vi "SavePanel.vi"(8 "error in":errorcluster) -> (0 "error out":errorcluster, 3 "Chaîne":string)   [LabVIEW 2019, in "PhotoLum.lvclass"]
uses:
  PhotoLum.lvclass
panel:
  in  "OtherMat":string caption="Matériaux (autres)"
  in  "Matériaux":u16(ring) items=["AlGaAs", "AlP", "GaAs", "GaN", "Ge", "InP", "Si", "SiGe", "Autres"]
  in  "unit":u16(ring) caption="Unités\nPre-amp." items=["mA/V", "µA/V", "nA/V", "pA/V"]
  in  "Facteur":u16(ring) caption="Facteur Pre-amp." items=["1", "2", "5", "10", "20", "50", "100", "200", "500"]
  in  "Preamp":u16(ring) caption="Pre-amplificateur" items=["Aucun", "SR570 Current Preamp", "SR560 Voltage Preamp"]
  in  "PLaser":dbl=1000.0 caption="Puissance(mW)" min=0.0 step=0.1 format="%#.1f"
  in  "Temp":dbl=1000.0 caption="Température(°K)" min=0.0 step=0.1 format="%#.1f"
  in  "Annuler":bool
  in  "Save":bool
  in  "Autres":string
  in  "Filtre":u16(ring) caption="Filtre Entrée" items=["Aucun", "Mauve", "Jaune 495nm", "Vert", "Orange", "Rouge 665nm", "Rouge 850nm", "SI"]
  in  "LN Cooled":bool
  in  "Échantillon":string
  in  "Excitation":u16(ring) caption="Source d'excitation" items=["HeCd 325nm", "Diode 532nm", "Diode 683nm", "Diode 786nm", "Diode 840nm", "Diode 905nm", "Diode 980nm"]
  in  "Détecteur":u16(ring) items=["PM Hamamatsu R9268", "Détecteur Ge EG&G", "Détecteur Si EG&G", "Détecteur InAs EG&G", "Détecteur InSb EG&G"]
  in  "Réseaux":u16(ring) items=["250nm", "1µm", "4µm", "8µm"]
  in  "2xInput":bool
  in  "OutputSlit":dbl caption="Largeur de fente de sortie (mm)"
  in  "SlitHeight":u16(ring) caption="Hauteur fente d'entrée" items=["2 cm", "1 cm", "2 mm", "Trou haut", "Trou centré", "Trou bas"]
  in  "InputSlit":dbl caption="Largeur de fente d'entrée (mm)"
  # "Paramètres du balayage"
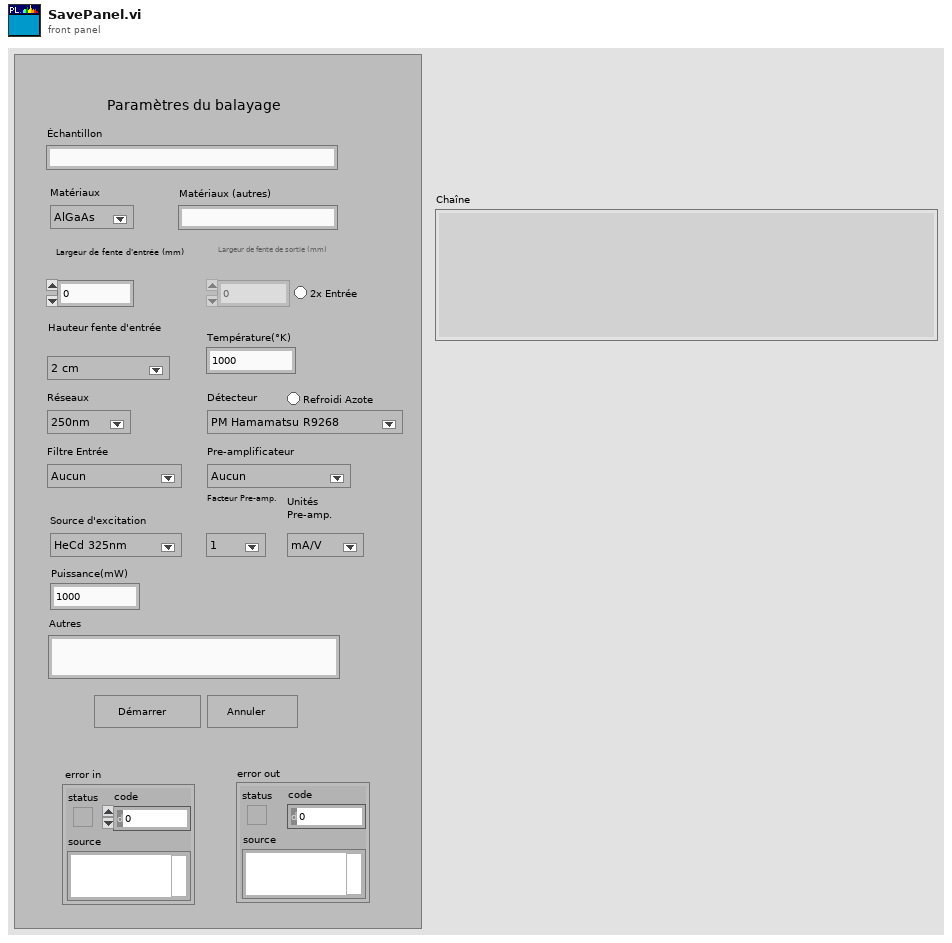
[diagram p1: front panel]
types:
  T1 = enum8{"Enabled", "Disabled", "Disabled and Grayed Out"}
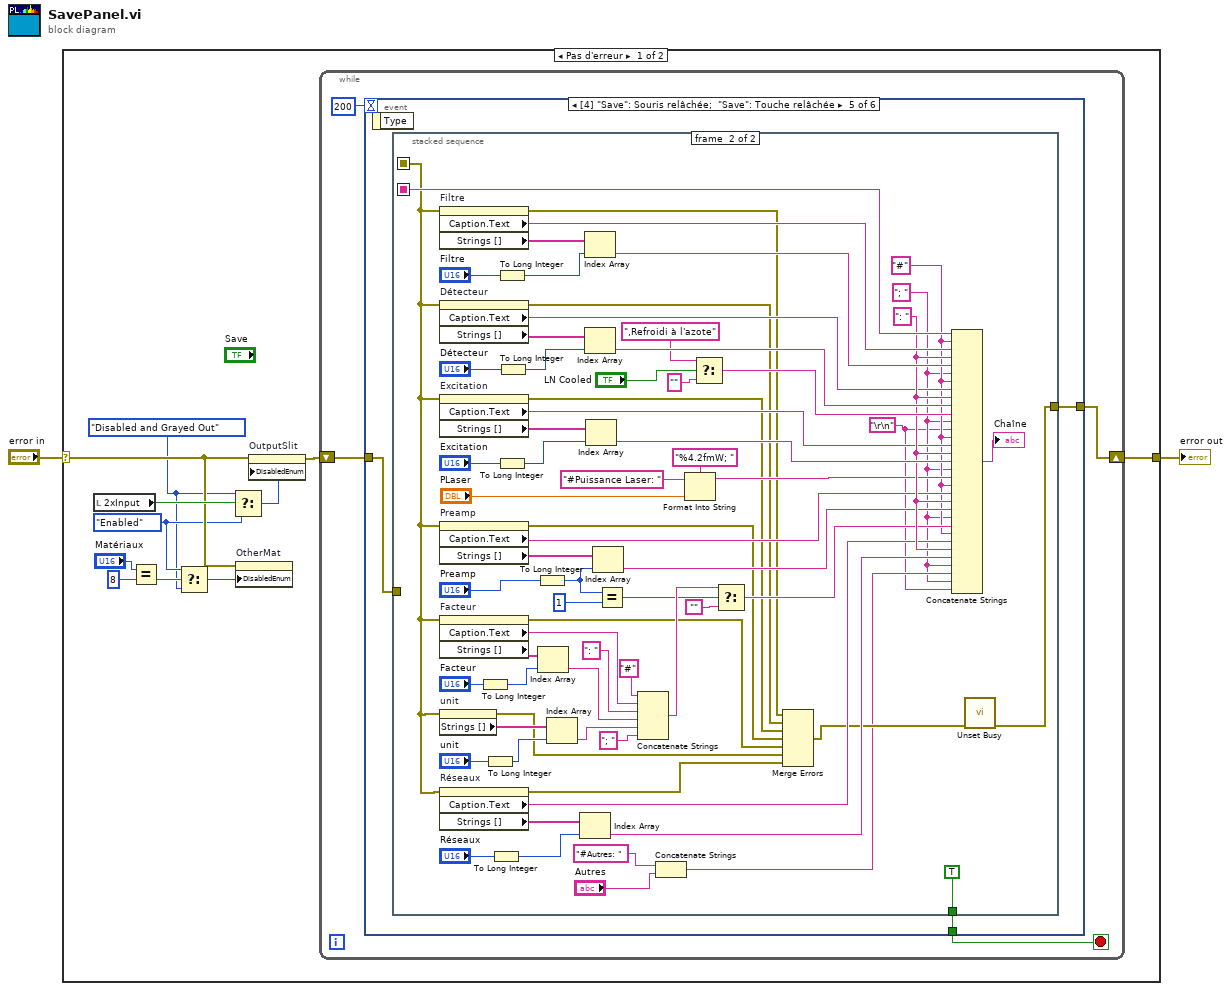
[diagram p0: block diagram]
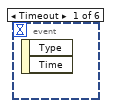
[diagram p2: hidden frame]
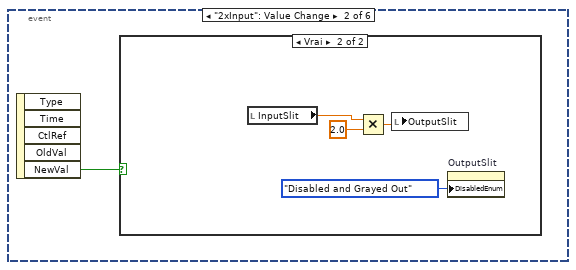
[diagram p3: hidden frame]
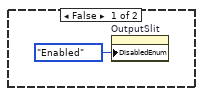
[diagram p4: hidden frame]
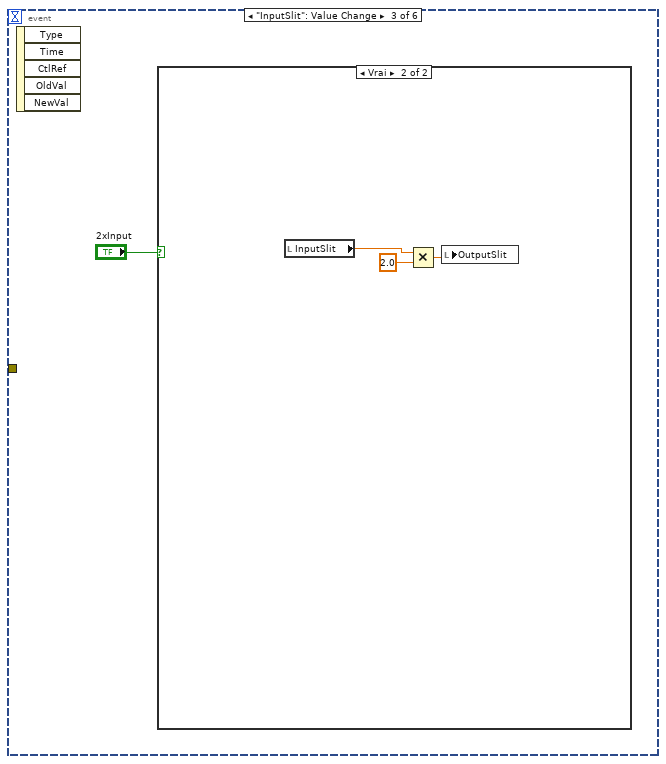
[diagram p5: hidden frame]
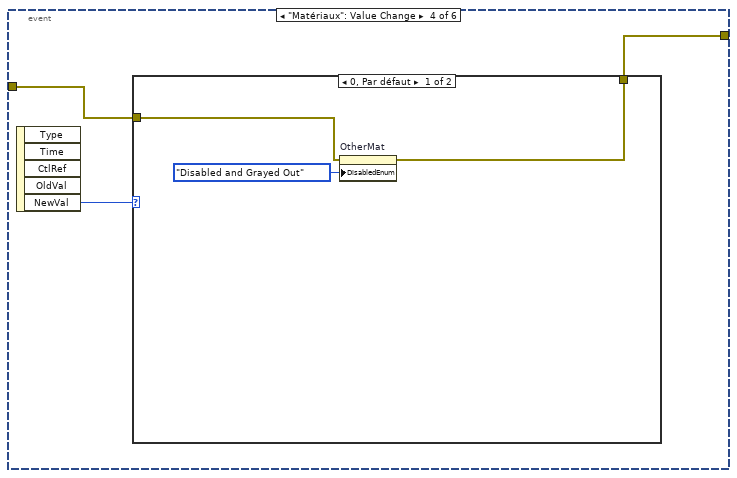
[diagram p7: hidden frame]
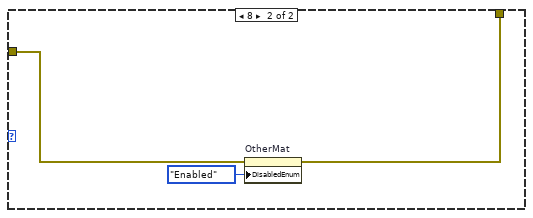
[diagram p8: hidden frame]
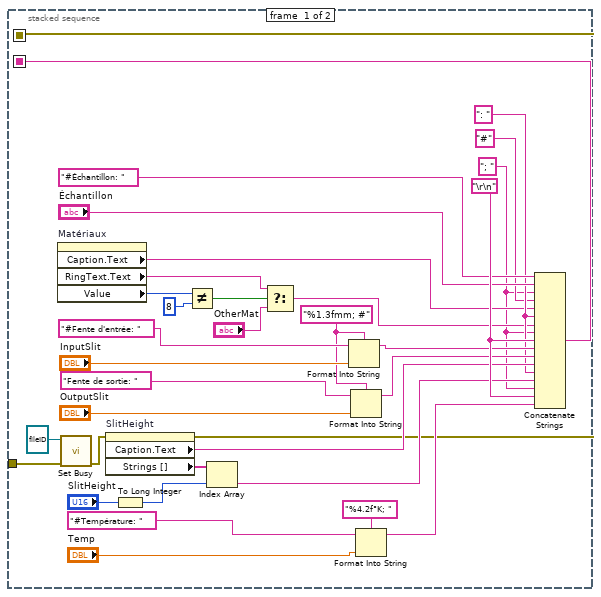
[diagram p9: hidden frame]
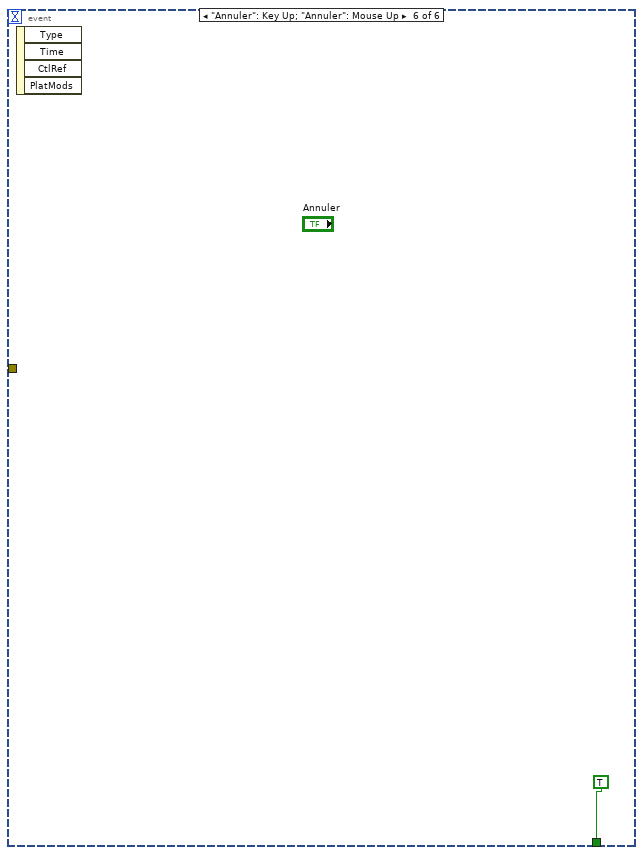
[diagram p10: hidden frame]
diagram:
  n1 = case shown="Pas d'erreur" "error in" {
    selector: "error in" -> [w9 w145]
    tunnel: [w13 w145] -> w2
    frame No Error {
      w4 = T1."Disabled and Grayed Out" ("Désactivé")
      w5 = T1."Enabled" ("Désactivé")
      n2 = local read "2xInput"() -> (w11:bool)
      n3 = Equal?(x="Matériaux", y=u16 8) -> (x = y?=w6:bool)
      n4 = Select(t=w5, s=w6, f=w4) -> (s? t:f=w3:T1)
      n5 = Select(t=w4, s=w11, f=w5) -> (s? t:f=w10:T1)
      n6 = property on="OtherMat" class="Ch"(error in=w9, "DisabledEnum"=w3) -> ()  [unwired: 1 in, 2 out]
      n7 = property on="OutputSlit" class="NumNb (strict)"(error in=w9, "DisabledEnum"=w10) -> (error out=w12:errorcluster)  [unwired: 1 in, 1 out]
      n8 = while {
        shift-right: [w14] -> w13
        shift-left: w12 -> [w15]
        stop <- w16 stop-if-true
        n9 = event shown="[4] \"Save\": Souris relâchée;  \"Save\": Touche relâchée" {
          selector: _ -> [_ _ _ _ _ _]
          dyn-events: _ -> [_ _ _ _ _ _]
          timeout: 200 -> [_ _ _ _ _ _]
          tunnel: [_ _ _ _ w39 TRUE] -> w16
          tunnel: w15 -> [_ _ _ w29 w38 _]
          tunnel: [_ _ _ w28 w37 _] -> w14
          event Timeout {
            n10 = event-data() -> ()  [unwired: 1 in, 2 out]
          }
          event "2xInput": Value Change {
            n11 = event-data() -> ("NewVal"=w18:bool)  [unwired: 1 in, 4 out]
            n12 = case shown="Vrai" w18 {
              frame False {
                n13 = property on="OutputSlit" class="NumNb (strict)"("DisabledEnum"=T1."Enabled" ("Désactivé")) -> ()  [unwired: 2 in, 2 out]
              }
              frame True {
                n14 = local read "InputSlit"() -> (w20:dbl)
                n15 = Multiply(x=w20, y=2.0) -> (x*y=w22:dbl)
                n16 = local write "OutputSlit"(w22) -> ()
                n17 = property on="OutputSlit" class="NumNb (strict)"("DisabledEnum"=T1."Disabled and Grayed Out" ("Désactivé")) -> ()  [unwired: 2 in, 2 out]
              }
            }
          }
          event "InputSlit": Value Change {
            n18 = event-data() -> ()  [unwired: 1 in, 5 out]
            n19 = case shown="Vrai" "2xInput" {
              frame False {
              }
              frame True {
                n20 = local read "InputSlit"() -> (w25:dbl)
                n21 = Multiply(x=w25, y=2.0) -> (x*y=w27:dbl)
                n22 = local write "OutputSlit"(w27) -> ()
              }
            }
          }
          event "Matériaux": Value Change {
            n23 = event-data() -> ("NewVal"=w30:u16)  [unwired: 1 in, 4 out]
            n24 = case shown="0, Par défaut" w30 {
              tunnel: w29 -> [w32 w35]
              tunnel: [w31 w34] -> w28
              frame 0, Default {
                n25 = property on="OtherMat" class="Ch"(error in=w32, "DisabledEnum"=T1."Disabled and Grayed Out" ("Désactivé")) -> (error out=w31:errorcluster)  [unwired: 1 in, 1 out]
              }
              frame 8 {
                n26 = property on="OtherMat" class="Ch"(error in=w35, "DisabledEnum"=T1."Enabled" ("Désactivé")) -> (error out=w34:errorcluster)  [unwired: 1 in, 1 out]
              }
            }
          }
          event "Save": Mouse Up; "Save": Key Up {
            n27 = event-data() -> ()  [unwired: 1 in, 1 out]
            n28 = stacked-sequence {
              seq-local: [w51 _] -> [_ w123]
              seq-local: [w50 _] -> [_ w81]
              tunnel: [_ TRUE] -> w39
              tunnel: w38 -> [w54 _]
              tunnel: [_ w79] -> w37
              frame #0 {
                w49 = ": " ("string")
                w64 = "%1.3fmm; #" ("chaîne de format")
                w73 = "\r\n"
                w40 = "; " ("chaîne")
                n29 = property on="Matériaux" class="MDér (strict)"() -> ("Caption.Text"=w47:string, "RingText.Text"=w43:string, "Value"=w45:u16)  [unwired: 2 in, 2 out]
                n30 = call <vilib>:"Set Busy.vi"("error in (no error)"=w54, "cursor ID"=refnum<k1> refnum) -> ("error out"=w53:errorcluster)  [unwired: 8 in, 1 out]
                n31 = property on="SlitHeight" class="MDér (strict)"(error in=w53) -> (error out=w50:errorcluster, "Caption.Text"=w60:string, "Strings []"=w63:string[])  [unwired: 1 in, 1 out]
                n32 = To Long Integer(number="SlitHeight") -> (32bit integer=w62:i32)
                n33 = Not Equal?(x=w45, y=u16 8) -> (x != y?=w44:bool)
                n34 = Index Array(array=w63, index=w62) -> (element=w59:string)
                n35 = Select(t=w43, s=w44, f="OtherMat") -> (s? t:f=w41:string)
                n36 = Format Into String(format string=w64, initial string="#Fente d'entrée: " ("chaîne"), "InputSlit") -> (resulting string=w68:string)  [unwired: 1 in, 1 out]
                n37 = Format Into String(format string=w64, initial string="Fente de sortie: " ("chaîne"), "OutputSlit") -> (resulting string=w67:string)  [unwired: 1 in, 1 out]
                n38 = Format Into String(format string="%4.2f°K; " ("chaîne de format"), initial string="#Température: " ("string"), "Temp") -> (resulting string=w55:string)  [unwired: 1 in, 1 out]
                n39 = Concatenate Strings("#Échantillon: " ("chaîne"), "Échantillon", w40, "#" ("string"), w47, w49, w41, w40, w73, w68, w67, w60, w49, w59, w40, w73, w55) -> (w51:string)
              }
              frame #1 {
                w89 = "#" ("chaîne")
                w74 = "\r\n"
                w75 = "; " ("chaîne")
                w120 = ": " ("chaîne")
                n40 = property on="Filtre" class="MDér (strict)"(error in=w81) -> (error out=w88:errorcluster, "Caption.Text"=w132:string, "Strings []"=w143:string[])  [unwired: 1 in, 1 out]
                n41 = property on="Détecteur" class="MDér (strict)"(error in=w81) -> (error out=w87:errorcluster, "Caption.Text"=w95:string, "Strings []"=w139:string[])  [unwired: 1 in, 1 out]
                n42 = property on="Excitation" class="MDér (strict)"(error in=w81) -> (error out=w86:errorcluster, "Caption.Text"=w92:string, "Strings []"=w135:string[])  [unwired: 1 in, 1 out]
                n43 = property on="Preamp" class="MDér (strict)"(error in=w81) -> (error out=w85:errorcluster, "Caption.Text"=w99:string, "Strings []"=w122:string[])  [unwired: 1 in, 1 out]
                n44 = property on="Facteur" class="MDér (strict)"(error in=w81) -> (error out=w84:errorcluster, "Caption.Text"=w103:string, "Strings []"=w110:string[])  [unwired: 1 in, 1 out]
                n45 = property on="unit" class="MDér (strict)"(error in=w81) -> (error out=w82:errorcluster, "Strings []"=w109:string[])  [unwired: 1 in, 1 out]
                n46 = property on="Réseaux" class="MDér (strict)"(error in=w81) -> (error out=w83:errorcluster, "Caption.Text"=w118:string, "Strings []"=w128:string[])  [unwired: 1 in, 1 out]
                n47 = To Long Integer(number="Facteur") -> (32bit integer=w106:i32)
                n48 = To Long Integer(number="unit") -> (32bit integer=w105:i32)
                n49 = To Long Integer(number="Réseaux") -> (32bit integer=w137:i32)
                n50 = To Long Integer(number="Filtre") -> (32bit integer=w141:i32)
                n51 = To Long Integer(number="Excitation") -> (32bit integer=w136:i32)
                n52 = To Long Integer(number="Détecteur") -> (32bit integer=w140:i32)
                n53 = To Long Integer(number="Preamp") -> (32bit integer=w114:i32)
                n54 = Index Array(array=w110, index=w106) -> (element=w101:string)
                n55 = Index Array(array=w109, index=w105) -> (element=w104:string)
                n56 = Index Array(array=w128, index=w137) -> (element=w96:string)
                n57 = Index Array(array=w143, index=w141) -> (element=w131:string)
                n58 = Index Array(array=w139, index=w140) -> (element=w130:string)
                n59 = Index Array(array=w135, index=w136) -> (element=w129:string)
                n60 = Index Array(array=w122, index=w114) -> (element=w119:string)
                n61 = Equal?(x=w114, y=1) -> (x = y?=w97:bool)
                n62 = Concatenate Strings("#" ("chaîne"), w103, ": " ("chaîne"), w101, w104, "; " ("chaîne")) -> (w98:string)
                n63 = Concatenate Strings("#Autres: " ("chaîne"), "Autres") -> (w76:string)
                n64 = Format Into String(format string="%4.2fmW; " ("chaîne de format"), initial string="#Puissance Laser: " ("string"), "PLaser") -> (resulting string=w115:string)  [unwired: 1 in, 1 out]
                n65 = Select(t=",Refroidi à l'azote" ("chaîne"), s="LN Cooled", f="" ("chaîne")) -> (s? t:f=w124:string)
                n66 = Select(t=w98, s=w97, f="") -> (s? t:f=w111:string)
                n67 = Merge Errors(w88, w87, w86, w85, w84, w82, w83) -> (w80:errorcluster)
                n68 = Concatenate Strings(w123, w89, w132, w120, w131, w75, w89, w95, w120, w130, w124, w75, w74, w89, w92, w120, w129, w75, w115, w89, w99, w120, w119, w75, w111, w89, w118, w120, w96, w75, w76, w75, w74) -> (→"Chaîne":string)
                n69 = call <vilib>:"Unset Busy.vi"("error in (no error)"=w80) -> ("error out"=w79:errorcluster)  [unwired: 10 in]
              }
            }
          }
          event "Annuler": Key Up; "Annuler": Mouse Up {
            n70 = event-data() -> ()  [unwired: 1 in, 4 out]
          }
        }
      }
    }
    frame Error {
    }
  }
  "error out" <- w2
